vi "SkidpadAttemptLEDWinker.vi"(6 "inputError":errorcluster, 8 "StateValue":T1, 9 "CurrentEntry":string, 10 "EventProgressDataInput":string[][](array[string]), 11 "inputRefOfLED":refnum<vi>[](array[refnum])) -> (0 "outputError":errorcluster)   [LabVIEW 2020]
uses:
  Control/SkidpadState.ctl
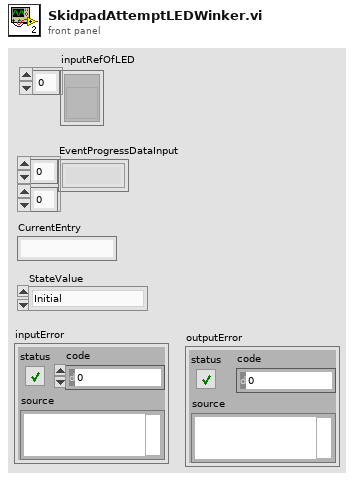
[diagram p1: front panel]
types:
  T1 = typedef "SkidpadState.ctl" = enum16{"Initial", "InputInfomation", "Ready", "1lap", "2lap", "3lap", "4lap", "FinshRunning", "LogRecord", "HardwareRelease", "WaittingforNext", "ProgramStop"}
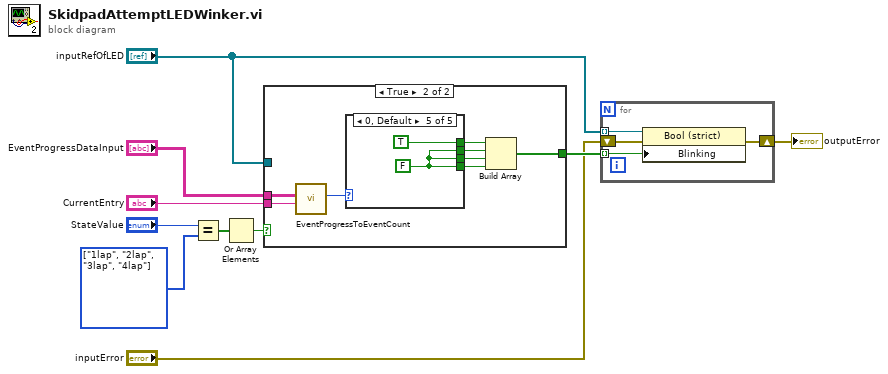
[diagram p0: block diagram]
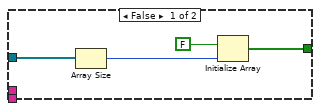
[diagram p2: hidden frame]
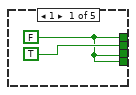
[diagram p3: hidden frame]
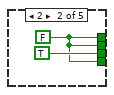
[diagram p4: hidden frame]
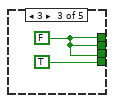
[diagram p5: hidden frame]
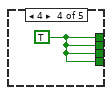
[diagram p6: hidden frame]
diagram:
  w3 = T1[] [enum."1lap", enum."2lap", enum."3lap", enum."4lap"] items=["Initial", "InputInfomation", "Ready", "1lap", "2lap", "3lap", "4lap", "FinshRunning", "LogRecord", "HardwareRelease", "WaittingforNext", "ProgramStop"]
  n1 = Equal?(x="StateValue", y=w3) -> (x = y?=w2:bool[])
  n2 = Or Array Elements(Boolean array=w2) -> (logical OR=w1:bool)
  n3 = case shown="True" w1 {
    tunnel: "inputRefOfLED" -> [w13 _]
    tunnel: "EventProgressDataInput" -> [_ w16]
    tunnel: "CurrentEntry" -> [_ w15]
    tunnel: [w10 w14] -> w7
    frame False {
      n4 = Array Size(array=w13) -> (size(s)=w12:i32)
      n5 = Initialize Array "Initialize Array"(FALSE, w12) -> (w10:bool[])
    }
    frame True {
      n6 = call "EventProgressToEventCount.vi"("CurrentEntry"=w15, "EventProgressDataInput"=w16) -> ("EventCount"=w17:i32)  [unwired: 9 in]
      n7 = case shown="0, Default" w17 {
        tunnel: [w22 w24 w26 w28 TRUE] -> w21
        tunnel: [TRUE w24 w26 w28 w29] -> w20
        tunnel: [w22 TRUE w26 w28 w29] -> w19
        tunnel: [w22 w24 TRUE w28 w29] -> w18
        frame 1 {
          w22 = FALSE
        }
        frame 2 {
          w24 = FALSE
        }
        frame 3 {
          w26 = FALSE
        }
        frame 4 {
          w28 = TRUE
        }
        frame 0, Default {
          w29 = FALSE
        }
      }
      n8 = Build Array "Build Array"(w21, w20, w19, w18) -> (w14:bool[])
    }
  }
  n9 = for {
    shift-right: [w33] -> _
    shift-left: _ -> [w34]
    tunnel: w7 -> [w32] mode=indexing
    tunnel: "inputRefOfLED" -> [w31] mode=indexing
    n10 = property class="Bool (strict)"(reference=w31, error in=w34, "Blinking"=w32) -> (error out=w33:errorcluster)  [unwired: 1 out]
  }
  "outputError" <- "inputError"
